vi "ReadString.vi"(8 "error in (no error)":errorcluster, 10 "Timeout":u32, 11 "TcpReader in":refnum<class "TcpReader.lvclass">) -> (0 "error out":errorcluster, 2 "String":string, 3 "TcpReader out":refnum<class "TcpReader.lvclass">)   [LabVIEW 2025, in "TcpReader.lvclass"]
doc: "Read data as a string from the TCP/IP connection"
uses:
  TcpReader.lvclass
  TcpReader.lvclass/TcpReader.ctl
  <userlib>/_OpenG.lib/error/error.llb/Filter Error Codes (Array)__ogtk.vi
  Interface/TCP/TCP/TCP.lvclass
  <userlib>/_OpenG.lib/error/error.llb/openg_error.lvlib
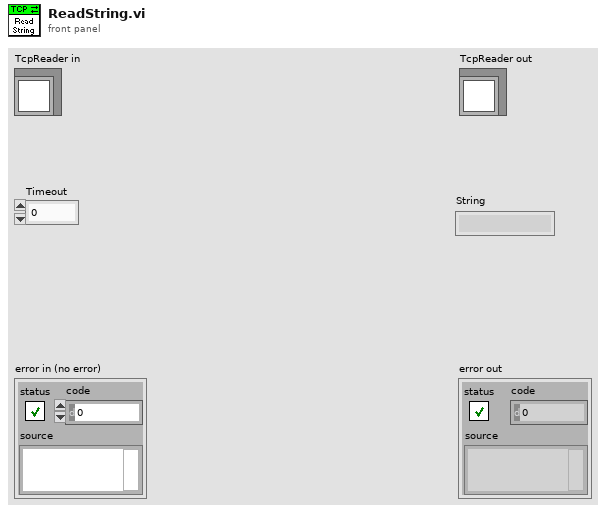
[diagram p1: front panel]
types:
  T1 = enum16{"Standard", "Buffered", "CRLF", "Immediate"}
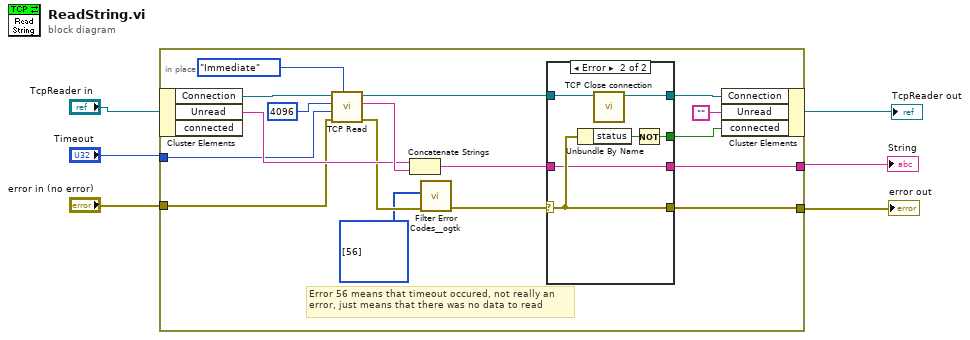
[diagram p0: block diagram]
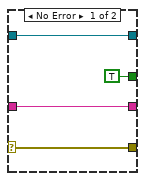
[diagram p2: hidden frame]
diagram:
  n1 = in-place "In Place Element Structure" {
    in-place-border: [w8] -> w1
    in-place-border: "error in (no error)" -> [w18]
    in-place-border: [w10] -> w3
    in-place-border: "Timeout" -> [w17]
    # "Error 56 means that timeout occured, not really an\nerror, just means that there was no data to read"
    n2 = in-place-cluster #1("TcpReader in") -> ("Connection"=w7:refnum<class "TCP.lvclass">, "Unread"=w20:string)  [unwired: 1 out]
    n3 = call-dynamic "TCP Read.vi"("mode (standard)"=T1."Immediate", "error in (no error)"=w18, "timeout ms (25000)"=w17, "bytes to read"=4096, "TCP in"=w7) -> ("error out"=w16:errorcluster, "data out"=w21:string, "TCP out"=w13:refnum<class "TCP.lvclass">)  [unwired: 4 in]
    n4 = Concatenate Strings(w20, w21) -> (w9:string)
    n5 = call-poly <userlib>:"Filter Error Codes__ogtk.vi"("Error In"=w16, "Error Codes to Filter"=i32[] [56]) -> ("Error Out"=w14:errorcluster)  [unwired: 7 in, 2 out]
    n6 = case shown="Error" w14 {
      selector: w14 -> [w25 w29]
      tunnel: w13 -> [w26 w33]
      tunnel: [w26 w32] -> w12
      tunnel: [TRUE w30] -> w11
      tunnel: [w25 w29] -> w10
      tunnel: [w24 w28] -> w8
      tunnel: w9 -> [w24 w28]
      frame No Error {
      }
      frame Error {
        n7 = Unbundle By Name(w29) -> ("status"=w31:bool)
        n8 = call-dynamic "TCP Close connection.vi"("TCP in"=w33) -> ("TCP out"=w32:refnum<class "TCP.lvclass">)  [unwired: 9 in, 1 out]
        n9 = Not(x=w31) -> (.not. x?=w30:bool)
      }
    }
    n10 = in-place-cluster #1("Connection"=w12, "Unread"="" ("Empty String Constant"), "connected"=w11) -> (→"TcpReader out":refnum<class "TcpReader.lvclass">)
  }
  "String" <- w1
  "error out" <- w3
